vi "GetSubMenuPosition.vi"(8 "error in (no error)":errorcluster, 10 "index":i32, 11 "menu in":refnum<class "menu.lvclass">) -> (0 "error out":errorcluster, 2 "position":cluster{"left":u32, "top":u32}, 3 "menu out":refnum<class "menu.lvclass">)   [LabVIEW 2009, in "menu.lvclass"]
uses:
  menu.lvclass
  menu.lvclass/menu.ctl
  Menu Item/menu item.lvclass
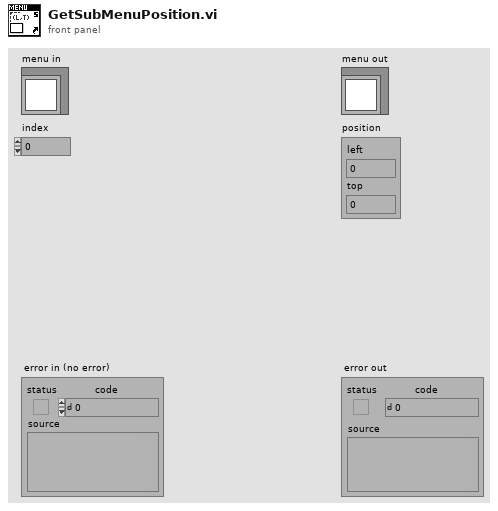
[diagram p1: front panel]
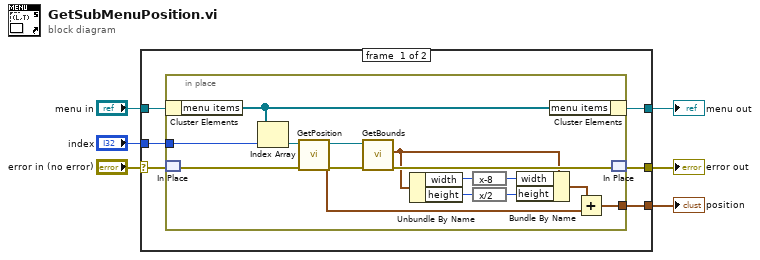
[diagram p0: block diagram]
diagram:
  n1 = case shown="No Error" "error in (no error)" {
    selector: "error in (no error)" -> [w10 w29]
    tunnel: [w9 w29] -> w3
    tunnel: [w8 w28] -> w5
    tunnel: "menu in" -> [w12 w28]
    tunnel: "index" -> [w11 _]
    tunnel: [w7 _] -> w1
    frame #0 {
      n2 = in-place {
        in-place-border: w11 -> [w26]
        in-place-border: [w15] -> w7
        n3 = in-place-cluster #1(w12) -> ("menu items"=w27:refnum<class "menu item.lvclass">[])
        n4 = in-place-match #2(w10) -> (w22:errorcluster)
        n5 = Index Array(array=w27, index=w26) -> (element=w25:refnum<class "menu item.lvclass">)
        n6 = call-dynamic "GetPosition.vi"("error in (no error)"=w22, "menu item in"=w25) -> ("error out"=w23:errorcluster, "position"=w17:cluster{"left":u32, "top":u32}, "menu item out"=w24:refnum<class "menu item.lvclass">)  [unwired: 7 in]
        n7 = call-dynamic "GetBounds.vi"("error in (no error)"=w23, "menu item in"=w24) -> ("error out"=w21:errorcluster, "bounds"=w20:cluster{"width":u32, "height":u32})  [unwired: 7 in, 1 out]
        n8 = Unbundle By Name(w20) -> ("width"=w14:u32, "height"=w19:u32)
        n9 = expression code="x-8"(w14) -> (w13:u32)
        n10 = expression code="x/2"(w19) -> (w18:u32)
        n11 = Bundle By Name(cluster=w20, "width"=w13, "height"=w18) -> (w16:cluster{"width":u32, "height":u32})
        n12 = in-place-cluster #1("menu items"=w27) -> (w8:refnum<class "menu.lvclass">)
        n13 = Add(x=w16, y=w17) -> (x+y=w15:cluster{u32, u32})
        n14 = in-place-match #2(w21) -> (w9:errorcluster)
      }
    }
    frame #1 {
    }
  }
  "menu out" <- w5
  "error out" <- w3
  "position" <- w1
